vi "Configure Trigger (PRunt).vi"(0 "VISA resource name":refnum<visa-resource-name>, 1 "Pulse Width Lower Limit (1E-6 s)":dbl=1e-06, 2 "Trigger Level Upper Limit (0)":dbl, 3 "Windows Type (0: TA)":i32(ring) items=["TA", "TB", "TAB"], 5 "Source (1: Channel 1)":i32(ring)=1 items=["Channel 1"=1, "Channel 2"=2, "Channel 3"=3, "Channel 4"=4], 7 "Polarity (0: Positive)":i32(ring) items=["Positive", "Negative", "Either"], 9 "Qualifier (0: None)":i32(ring) items=["None", "Greater", "Less", "InRange"], 11 "error in (no error)":errorcluster, 12 "Pulse Width Upper Limit (2E-6)":dbl=2e-06, 13 "Trigger Level Lower Limit (0)":dbl) -> (4 "VISA resource name out":refnum<visa-resource-name>, 15 "error out":errorcluster)   [LabVIEW 2015, in "ZhiYuan ZDS Series for TCP.lvlib"]
doc: "Configures the setting for runt trigger.\n\nNote: This VI is only applicable for DS 2000 Series."
uses:
  ZhiYuan ZDS Series for TCP.lvlib
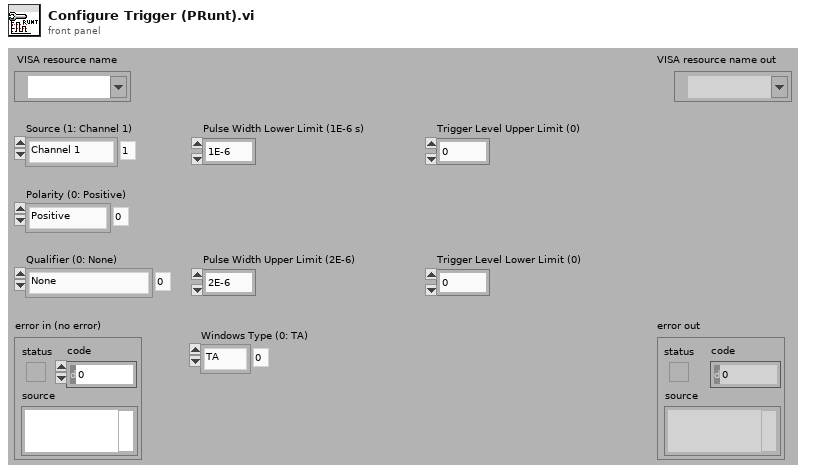
[diagram p1: front panel]
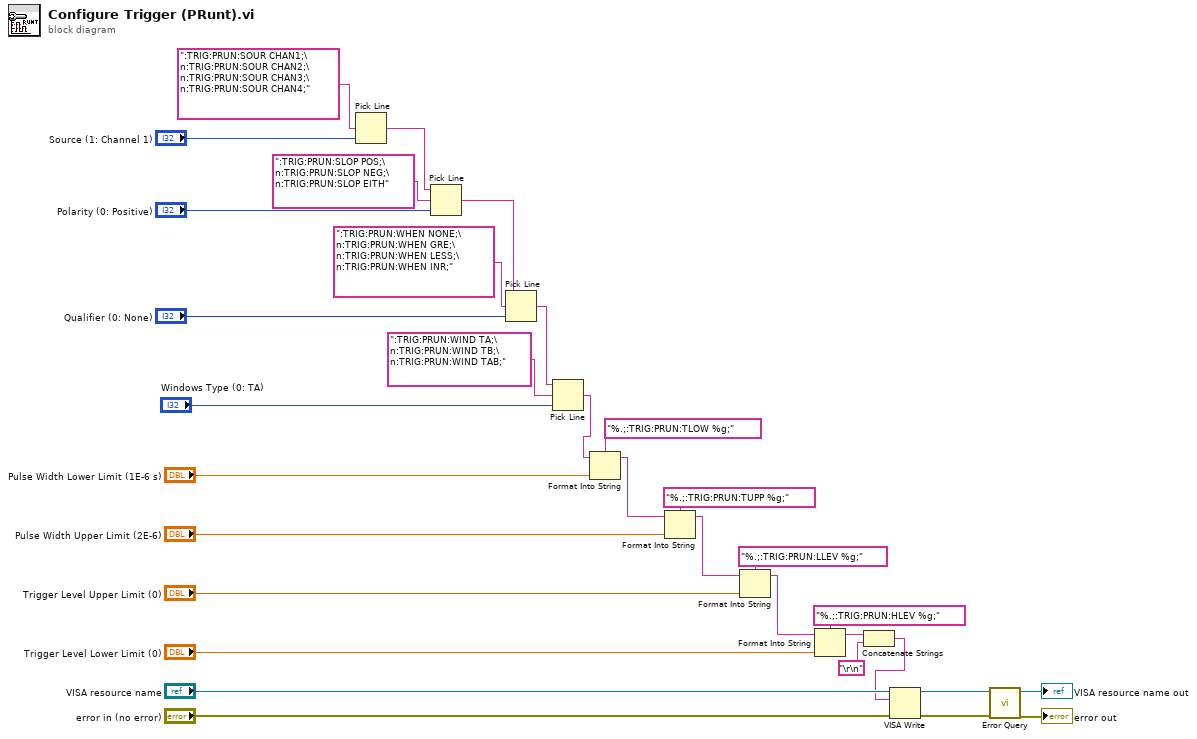
[diagram p0: block diagram]
diagram:
  n1 = Pick Line(multi-line string=":TRIG:PRUN:SOUR CHAN1;\n:TRIG:PRUN:SOUR CHAN2;\n:TRIG:PRUN:SOUR CHAN3;\n:TRIG:PRUN:SOUR CHAN4;", line index="Source (1: Channel 1)") -> (output string=w28:string)  [unwired: 1 in]
  n2 = Pick Line(string ("")=w28, multi-line string=":TRIG:PRUN:SLOP POS;\n:TRIG:PRUN:SLOP NEG;\n:TRIG:PRUN:SLOP EITH", line index="Polarity (0: Positive)") -> (output string=w25:string)
  n3 = Pick Line(string ("")=w25, multi-line string=":TRIG:PRUN:WHEN NONE;\n:TRIG:PRUN:WHEN GRE;\n:TRIG:PRUN:WHEN LESS;\n:TRIG:PRUN:WHEN INR;", line index="Qualifier (0: None)") -> (output string=w7:string)
  n4 = Pick Line(string ("")=w7, multi-line string=":TRIG:PRUN:WIND TA;\n:TRIG:PRUN:WIND TB;\n:TRIG:PRUN:WIND TAB;", line index="Windows Type (0: TA)") -> (output string=w4:string)
  n5 = Format Into String(format string="%.;:TRIG:PRUN:TLOW %g;", initial string=w4, "Pulse Width Lower Limit (1E-6 s)") -> (resulting string=w22:string)  [unwired: 1 in, 1 out]
  n6 = Format Into String(format string="%.;:TRIG:PRUN:TUPP %g;", initial string=w22, "Pulse Width Upper Limit (2E-6)") -> (resulting string=w19:string)  [unwired: 1 in, 1 out]
  n7 = Format Into String(format string="%.;:TRIG:PRUN:LLEV %g;", initial string=w19, "Trigger Level Upper Limit (0)") -> (resulting string=w16:string)  [unwired: 1 in, 1 out]
  n8 = Format Into String(format string="%.;:TRIG:PRUN:HLEV %g;", initial string=w16, "Trigger Level Lower Limit (0)") -> (resulting string=w3:string)  [unwired: 1 in, 1 out]
  n9 = Concatenate Strings(w3, "\r\n") -> (w1:string)
  n10 = VISA Write(VISA resource name="VISA resource name", write buffer=w1, error in (no error)="error in (no error)") -> (VISA resource name out=w11:refnum<visa-resource-name>, error out=w10:errorcluster)  [unwired: 1 out]
  n11 = call "Error Query.vi"("error in (no error)"=w10, "VISA resource name"=w11) -> ("error out"=→"error out":errorcluster, "VISA resource name out"=→"VISA resource name out":refnum<visa-resource-name>)  [unwired: 6 in, 2 out]
